vi "QVA_DeleteVariantAttribute.vi"(0 "QueueIn":refnum<queue>, 1 "Name":string, 5 "ErrorIn":errorcluster, 9 "Timeout":i32=-1) -> (14 "QueueOut":refnum<queue>, 16 "Timeout":bool, 17 "FoundAndRemoved":bool, 19 "ErrorOut":errorcluster)   [LabVIEW 2016]
doc: "Löscht ein Variant Attribute aus dem QVA\n\nsige / 3.12.13"
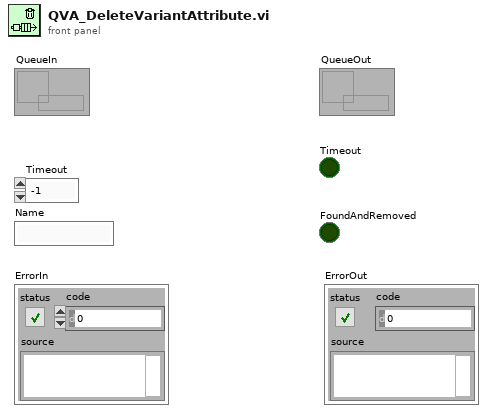
[diagram p1: front panel]
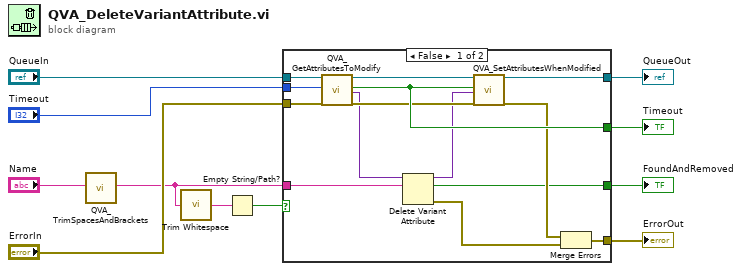
[diagram p0: block diagram]
diagram:
  n1 = call "QVA_TrimSpacesAndBrackets.vi"("String"="Name") -> ("TrimmedString"=w1:string)  [unwired: 18 in]
  n2 = call <vilib>:"Trim Whitespace.vi"("string"=w1) -> ("trimmed string"=w3:string)  [unwired: 1 in]
  n3 = Empty String/Path?(string/path=w3) -> (empty?=w2:bool)
  n4 = case shown="False" w2 {
    tunnel: "QueueIn" -> [w24 w27]
    tunnel: "Timeout" -> [w23 _]
    tunnel: "ErrorIn" -> [w22 w26]
    tunnel: [w21 _] -> w8
    tunnel: [w20 w27] -> w7
    tunnel: [w17 w26] -> w6
    tunnel: [w14 _] -> w5
    tunnel: w1 -> [w13 _]
    frame False {
      n5 = call "QVA_GetAttributesToModify.vi"("QueueIn"=w24, "Timeout"=w23, "ErrorIn"=w22) -> ("QueueOut"=w25:refnum<queue>, "Timeout"=w21:bool, "VariantData"=w16:variant, "ErrorOut"=w18:errorcluster)  [unwired: 13 in]
      n6 = Delete Variant Attribute(6:w13, 7:w16) -> (0:w12:errorcluster, 2:w14:bool, 3:w15:variant)  [unwired: 1 in]
      n7 = call "QVA_SetAttributesWhenModified.vi"("QueueIn"=w25, "SkipAfterTimeout"=w21, "VariantData"=w15, "ErrorIn"=w18) -> ("QueueOut"=w20:refnum<queue>, "ErrorOut"=w19:errorcluster)  [unwired: 14 in]
      n8 = Merge Errors(w19, w12) -> (w17:errorcluster)
    }
    frame True {
    }
  }
  "QueueOut" <- w7
  "ErrorOut" <- w6
  "Timeout" <- w8
  "FoundAndRemoved" <- w5
